vi "Write Data Test.vi"(8 "error in (no error)":errorcluster caption="entrée d'erreur (pas d'erreur)", 11 "Database Altyor en entrée":refnum<class "Database Altyor Packaging.lvclass">) -> (0 "error out":errorcluster caption="sortie d'erreur", 3 "Database Altyor en sortie":refnum<class "Database Altyor Packaging.lvclass">)   [LabVIEW 2020, in "Library Instrument & Equipement.lvlib" / "Library Database.lvlib" / "Database Altyor Packaging.lvclass"]
uses:
  Database Altyor Packaging.lvclass
  C:/Users/ngarcin/OneDrive - Altyor/Standard TB/Suite TB45/Class/Database/Database drivers/Database Drivers.lvclass
  Commun VI/TypeDef/Variable Printable.ctl
  Commun VI/Library Commun.lvlib
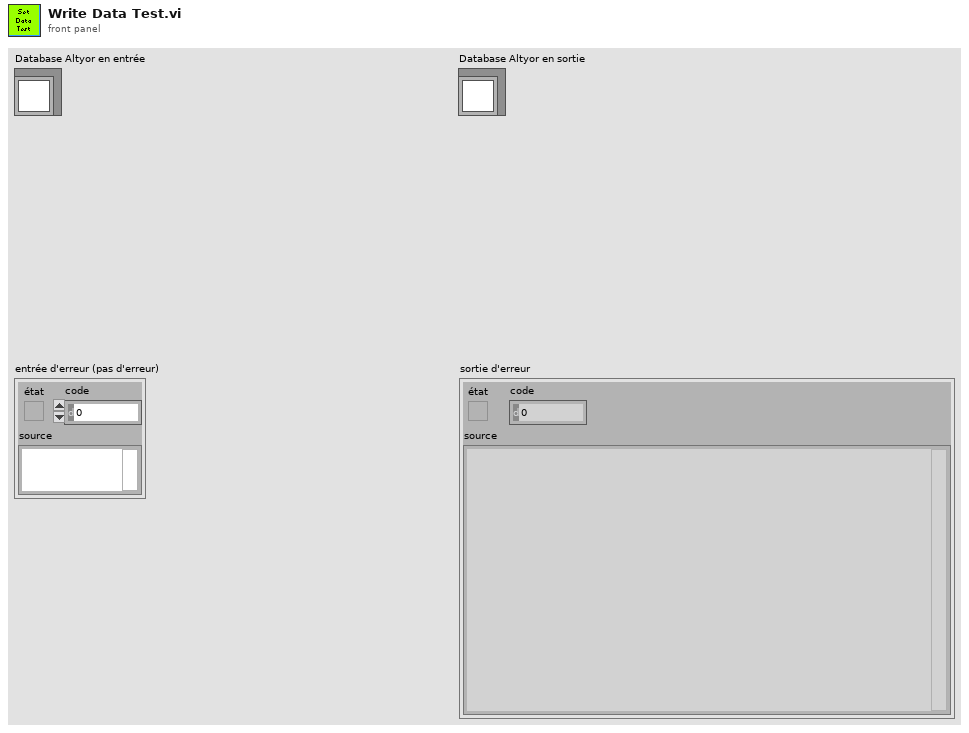
[diagram p1: front panel]
types:
  T1 = typedef "Variable Printable.ctl" = string
  T2 = enum16{"Get Variable", "Get All Variables", "Set Variable", "Delete Variable", "Delete All Variable"}
  T3 = cluster{"Key_Test":u32, "idPackaging":u32, "Name":string, "Name":string, "SerialNumber":string}
  T4 = cluster{"Key_Test":u32, "idPackaging":u32, "Name":string, "Name":string, "SerialNumber":string}[]
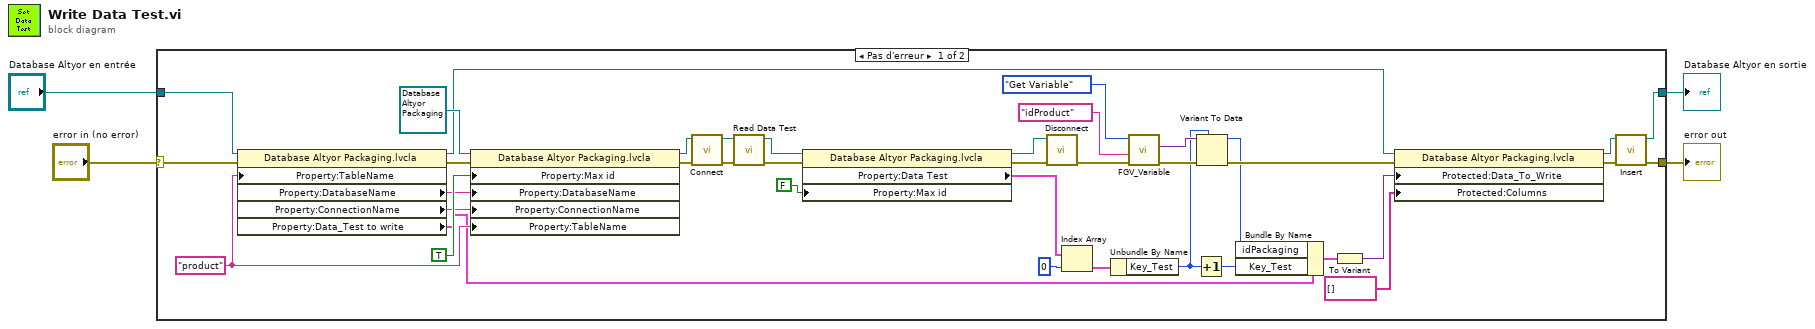
[diagram p0: block diagram]
diagram:
  n1 = case shown="Pas d'erreur" "error in (no error)" {
    selector: "error in (no error)" -> [w37 w44]
    tunnel: [w39 w44] -> w2
    tunnel: [w40 w43] -> w1
    tunnel: "Database Altyor en entrée" -> [w38 w43]
    frame No Error {
      w7 = "product" ("TableName")
      n2 = property class="Database Altyor Packaging.lvcla"(reference=w38, error in=w37, "Property:TableName"=w7) -> (reference out=w11:refnum<class "Database Altyor Packaging.lvclass">, error out=w35:errorcluster, "Property:DatabaseName"=w8:string, "Property:ConnectionName"=w9:string, "Property:Data_Test to write"=w6:T3)
      n3 = property class="Database Altyor Packaging.lvcla"(reference=refnum<class "Database Altyor Packaging.lvclass"> refnum ("Library Database.lvlib:Database Altyor.lvclass"), error in=w35, "Property:Max id"=TRUE ("Max id"), "Property:DatabaseName"=w8, "Property:ConnectionName"=w9, "Property:TableName"=w7) -> (reference out=w17:refnum<class "Database Altyor Packaging.lvclass">, error out=w14:errorcluster)
      n4 = call-dynamic "Connect.vi"("error in (no error)"=w14, "Database Altyor en entrée"=w17) -> ("error out"=w15:errorcluster, "Database Altyor en sortie"=w16:refnum<class "Database Altyor Packaging.lvclass">)  [unwired: 8 in]
      n5 = call-dynamic "Read Data Test.vi"("error in (no error)"=w15, "Database Altyor en entrée"=w16) -> ("error out"=w21:errorcluster, "Database Altyor en sortie"=w20:refnum<class "Database Altyor Packaging.lvclass">)  [unwired: 8 in]
      n6 = property class="Database Altyor Packaging.lvcla"(reference=w20, error in=w21, "Property:Max id"=FALSE ("Max id")) -> (reference out=w13:refnum<class "Database Altyor Packaging.lvclass">, error out=w12:errorcluster, "Property:Data Test"=w5:T4)
      n7 = call-dynamic "Disconnect.vi"("error in (no error)"=w12, "Database Altyor en entrée"=w13) -> ("error out"=w10:errorcluster)  [unwired: 8 in, 1 out]
      n8 = Index Array(array=w5, index=0 ("indice")) -> (element=w34:T3)
      n9 = Unbundle By Name(w34) -> ("Key_Test"=w24:u32)
      n10 = call "FGV_Variable.vi"("error in (no error)"=w10, "Variable"=T1 "idProduct", "Function"=T2."Get Variable") -> ("error out"=w28:errorcluster, "Data Out"=w25:variant)  [unwired: 6 in, 1 out]
      n11 = Increment(x=w24) -> (x+1=w29:u32)
      n12 = Variant To Data(error in=w28, type=w24, Variant=w25) -> (data=w23:u32, error out=w26:errorcluster)
      n13 = Bundle By Name(cluster=w6, "idPackaging"=w23, "Key_Test"=w29) -> (w32:T3)
      n14 = To Variant(anything=w32) -> (Variant=w36:variant)
      n15 = property class="Database Altyor Packaging.lvcla"(reference=w11, error in=w26, "Protected:Data_To_Write"=w36, "Protected:Columns"=string[] [] ("Columns")) -> (reference out=w42:refnum<class "Database Altyor Packaging.lvclass">, error out=w41:errorcluster)
      n16 = call-dynamic "Insert.vi"("error in (no error)"=w41, "Database Drivers en entrée"=w42) -> ("error out"=w39:errorcluster, "Database Drivers en sortie"=w40:refnum<class "Database Altyor Packaging.lvclass">)  [unwired: 8 in]
    }
    frame Error {
    }
  }
  "error out" <- w2
  "Database Altyor en sortie" <- w1
